vi "ApplicationGlobal.vi"() -> ()   [LabVIEW 2016]
uses:
  Tools/Windows/Windows.ExitAction.ctl
panel:
  in  "ResultsPathIgnored":path=path "D:/svn/LineTraceSystem/SOFTWARE/logs/results"
  in  "ResultsPathError":path=path "D:/svn/LineTraceSystem/SOFTWARE/logs/results"
  in  "ResultsPathExported":path=path "D:/svn/LineTraceSystem/SOFTWARE/logs/results"
  in  "ProductResultsPath":path=path "D:/svn/LineTraceSystem/SOFTWARE/logs/results"
  in  "VariantsPath":path=path "C:/SOFTWARE/settings/variants"
  in  "ResultsPath":path=path "D:/svn/LineTraceSystem/SOFTWARE/logs/results"
  out "Unlock":bool
  in  "font colors":u32[](array[colorbox])=[0, 0, 0, 0, 0, 0, 0, 16448250, 0, 0, 13816530]
  in  "status colors":u32[](array[colorbox])=[16777225, 16775210, 16759552, 9868950, 7864153, 16744576, 8454143, 16711680, 16744640, 16744640, 13816530]
  out "UnconfirmedError":bool
  in  "EventPath":path=path "C:/SOFTWARE/logs/events"
  out "AppDate-PC":string
  in  "Status":string
  in  "ExitAction":T1=enum."Shut Down PC"
  out "AppName-PC":string
  out "Changelog":string
  out "AppVer-PC":string
  out "Quitting":bool
  in  "LogPath":path=path "C:/SOFTWARE/logs"
  in  "SettingsPath":path=path "D:/svn/LineTraceSystem/SOFTWARE/settings"
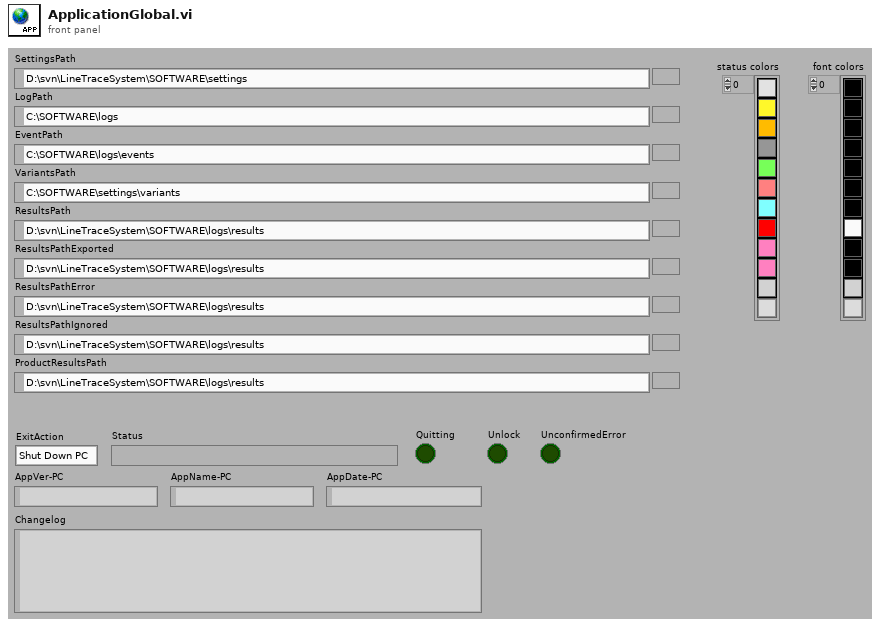
[diagram p1: front panel]
types:
  T1 = typedef "Windows.ExitAction.ctl" = enum16{"Log off from PC", "Shut Down PC", "Reboot PC", "Close Program"}
diagram:
